vi "Table, Get Column Value, Double.vi"(0 "error in":errorcluster, 3 "Tbl Refnum":refnum<vi>, 4 "column (0)":i32) -> (7 "error out":errorcluster, 9 "Value":dbl[](array[numeric]), 10 "Tbl Refnum out":refnum<vi>)   [LabVIEW 2010]
doc: "This function gets a single column of double precision numeric values from a table."
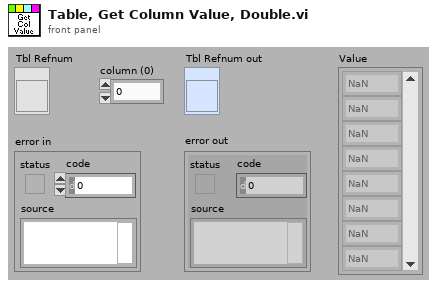
[diagram p1: front panel]
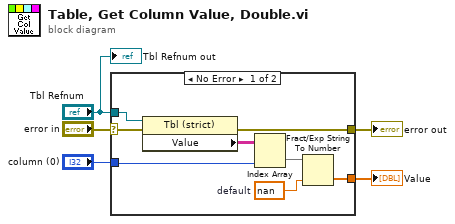
[diagram p0: block diagram]
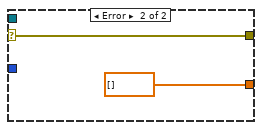
[diagram p2: hidden frame]
diagram:
  n1 = case shown="No Error" "error in" {
    selector: "error in" -> [w12 w15]
    tunnel: "Tbl Refnum" -> [w13 _]
    tunnel: [w9 w15] -> w5
    tunnel: "column (0)" -> [w10 _]
    tunnel: [w6 dbl[] []] -> w1
    frame No Error {
      w7 = nan  # default
      n2 = property class="Tbl (strict)"(reference=w13, error in=w12) -> (error out=w9:errorcluster, "Value"=w11:string[][])  [unwired: 1 out]
      n3 = Index Array(array=w11, index (col)=w10) -> (element=w8:string[])  [unwired: 1 in]
      n4 = Fract/Exp String To Number(string=w8, default (0 dbl)=w7) -> (number=w6:dbl[])  [unwired: 2 in, 1 out]
    }
    frame Error {
    }
  }
  "error out" <- w5
  "Value" <- w1
  "Tbl Refnum out" <- "Tbl Refnum"
